vi "Read Components Notifier.vi"(8 "error in (no error)":errorcluster, 11 "Item Ref in":T1 format="%.0x") -> (0 "error out":errorcluster, 2 "Components":refnum<class "Component.lvclass">[](array[class]), 3 "Item Ref out":T1 format="%.0x")   [LabVIEW 2017, in "DSF System Explorer.lvlib"]
uses:
  DSF System Explorer.lvlib
  <vilib>/NI Veristand/Custom Device API/Custom Device Item Ref.ctl
  DSF Core.lvlibp/Classes/Component/Component.lvclass
  <vilib>/NI Veristand/Custom Device API/Custom Device API.lvlib
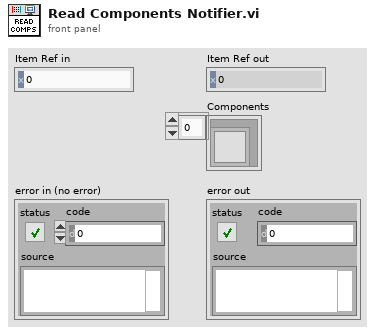
[diagram p1: front panel]
types:
  T1 = typedef "Custom Device API.lvlib/Custom Device Item Ref.ctl" = u64
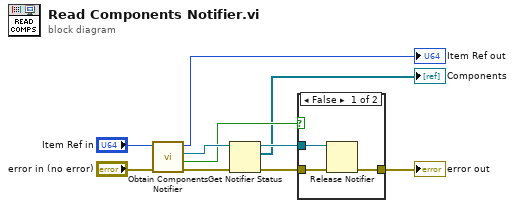
[diagram p0: block diagram]
diagram:
  n1 = call "Obtain Components Notifier.vi"("error in (no error)"="error in (no error)", "Item Ref in"="Item Ref in") -> ("error out"=w5:errorcluster, "created new?"=w2:bool, "comps notifier"=w9:refnum<notifier>, "Item Ref out"=→"Item Ref out":T1)  [unwired: 6 in]
  n2 = Get Notifier Status(notifier=w9, error in (no error)=w5) -> (notifier out=w6:refnum<notifier>, current notification=→"Components":refnum<class "Component.lvclass">[], error out=w10:errorcluster)  [unwired: 2 out]
  n3 = case shown="False" w2 {
    tunnel: w10 -> [w13 w14]
    tunnel: w6 -> [w12 _]
    tunnel: [w11 w14] -> w7
    frame False {
      n4 = Release Notifier(notifier=w12, error in (no error)=w13) -> (error out=w11:errorcluster)  [unwired: 1 in, 2 out]
    }
    frame True {
    }
  }
  "error out" <- w7
